vi "ADC INL_sweep_working_new.vi"(8 "error in (no error)":errorcluster, 9 "Sequence parameters":string[][](array[string])=[["Min limit", "Max limit", "Register sheet file", "Register Sheet"], ["", "", "CC2600.xls", "TX_BLE;Trim"], ["Reg write (addr;value)", "Operating frequency [Hz]", "", ""], ["NA", "2.44G", "", ""]], 10 "Run type":i32, 11 "Method parameters":T4={"Dev"={"Do not disturb DUT"=FALSE, "XOSC"=32000000.0, "Board type"="", "EM"="", "Configure tempboard"=TRUE, "Device specific info"=[], "Generic Object"=refnum}, "Method"={"Run type"=1, "Test name"="Current LPM2 4", "Comment"="", "Results folder"="", "AFC"=enum."Off", "Method name"="Current LPM2 4", "Method results"={"Excel brief report"=FALSE, "Spotfire report"=FALSE, "Starfish report"=FALSE}, "Operator"="", "Reference time"=timestamp(0 s since 1904-01-01), "AFC delay"=0.0, "Initialization"=enum."Enabled", "MD5 Sum"="", "HW addon board"=enum."None", "AFC Regsheet"="", "AFC Regfile"=path "", "dummy"=0.0}, "Inst"={"Instr"={"PS1"={"Name"="", "GPIB address"="", "VISA session"=""}, "PS2"={"Name"="", "GPIB address"="", "VISA session"=""}, "TC1"={"Name"="", "GPIB address"="", "VISA session"=""}, "TC2"={"Name"="", "GPIB address"="", "VISA session"=""}, "SA1"={"Name"="", "GPIB address"="", "VISA session"=""}, "SA2"={"Name"="", "GPIB address"="", "VISA session"=""}, "SG1"={"Name"="", "GPIB address"="", "VISA session"=""}, "SG2"={"Name"="", "GPIB address"="", "VISA session"=""}, "SG3"={"Name"="", "GPIB address"="", "VISA session"=""}, "MI1"={"Name"="", "GPIB address"="", "VISA session"=""}, "MI2"={"Name"="", "GPIB address"="", "VISA session"=""}, "SW SA"={"Name"="", "Controller addr"=""}, "SW SG"={"Name"="", "Controller addr"=""}, "MI3"={"Name"="", "GPIB address"="", "VISA session"=""}}, "Switchbox"={"RF Path"=0, "Cal compensation"=enum."TX", "Switchbox gain mode"="", "State"=enum."TX"}, "Instr to control (i.e. SA1)"="Default", "Intrument info string"=""}, "Sequence parameters"=[["Weight", "Min Limit", "Max Limit", "Register Sheet", "", "", "", "", "", "", "", "", ""], ["Vital", "", "1", "LPM2", "", "", "", "", "", "", "", "", ""], ["Resolution", "Reg write (addr;value)", "Chip mode", "Range", "", "", "", "", "", "", "", "", ""], ["u", "NA", "", "auto", "", "", "", "", "", "", "", "", ""]], "Cond"={"Temp logged"=25.0, "VDD1_PS1_6V"=-999.0, "VDD2_PS1_25V"=-999.0, "VDD4_PS2_25V"=-999.0, "VDD3_PS2_6V"=-999.0}, "Meas config"={"X-axis inner loop index"=32000000, "Y-axis outer loop index"=32000000, "X-axis"=[], "Y-axis"=[], "X-axis array req size"=32000000, "Y-axis array req size"=32000000, "Param description"=[], "Use meas clust for reporting"=FALSE, "Parameter index (page)"=0, "X-axis name"="", "Y-axis name"=""}} {"Cond"."VDD3_PS2_6V" format="%.3f"; "Cond"."VDD4_PS2_25V" format="%.3f"; "Cond"."VDD2_PS1_25V" format="%.3f"; "Cond"."VDD1_PS1_6V" format="%.3f"; "Method"."dummy" format="%.1p"; "Method"."AFC delay" format="%.1p"; "Dev"."XOSC" format="%.3p"}) -> (0 "error out":errorcluster, 1 "End method error":T3, 2 "Short Results":string[](array[string])=["0.00", "0.00", "0.00", "0.00"], 3 "Result summary":string[][](array[string])=[["Critical", "Output Power@2405 MHz", "-3", "4", "dBm"], ["Critical", "Output Power@2410 MHz", "-3", "4", "dBm"]])   [LabVIEW 2019]
doc: "[AutoDocStart]Performs crystal accuracy measurements. Measures the offset from ideal frequency. Primarily used for tuning XOSC capacitors and verifying XOSC trims.\n\nSweeping parameters: operating frequency, OSC override value and VDDR level\n\nResults: Offset frequency in ppm[AutoDocEnd]"
uses:
  User Lib/Utilities/Cluster definitions/Method input.ctl
  User Lib/Utilities/Cluster definitions/Device specific info.ctl
  User Lib/Utilities/Controls/Automatic Frequency Compensation types.ctl
  User Lib/Utilities/Controls/Method Reports.ctl
  User Lib/Utilities/Cluster definitions/Method Initialization.ctl
  User Lib/Utilities/Controls/HW addon boards.ctl
  User Lib/Utilities/Cluster definitions/Instr clust.ctl
  User Lib/Utilities/Switchbox control/SwitchBox_State._ENUMctl.ctl
  User Lib/Utilities/Cluster definitions/End method error cluster.ctl
  User Lib/Utilities/Cluster definitions/DUT vdd control.ctl
  User Lib/Utilities/Cluster definitions/DUT VDD4.ctl
  User Lib/Utilities/Cluster definitions/DUT VDD3.ctl
  User Lib/Utilities/Cluster definitions/DUT VDD2.ctl
  User Lib/Utilities/Cluster definitions/DUT VDD1.ctl
  ad5dbd7b-cdfb-4125-adc4-1165e2874c87.vi
  3f8b4189-43b3-45b7-8bba-bb7e10ae7045.vi
  42f514b6-df04-40b6-a03b-a487344522a2.vi
  dbdc58e7-b514-4632-b463-1ba2de0afab7.vi
  5201a9fb-abbc-4d1d-b83d-08253667edc6.vi
panel:
  out "output cluster 8":T1={"Average Hits \nper Code "=198.76479217603912, "Min DNL"=-0.30764433555407467, "Min INL"=-0.5231398172109945, "Max INL"=0.7801825995135989, "Max DNL"=0.8022935268616486, "DNL Range"=0.5549689312078616, "INL Range"=0.6516612083622967}
  out "ADC samples 8":u32[](array[numeric])
  out "output cluster 7":T1={"Average Hits \nper Code "=198.76479217603912, "Min DNL"=-0.30764433555407467, "Min INL"=-0.5231398172109945, "Max INL"=0.7801825995135989, "Max DNL"=0.8022935268616486, "DNL Range"=0.5549689312078616, "INL Range"=0.6516612083622967}
  out "ADC samples 7":u32[](array[numeric])
  out "output cluster 5":T1={"Average Hits \nper Code "=198.76479217603912, "Min DNL"=-0.30764433555407467, "Min INL"=-0.5231398172109945, "Max INL"=0.7801825995135989, "Max DNL"=0.8022935268616486, "DNL Range"=0.5549689312078616, "INL Range"=0.6516612083622967}
  out "ADC samples 5":u32[](array[numeric])
  in  "Tab Control":T2(tab)
  # "°C"
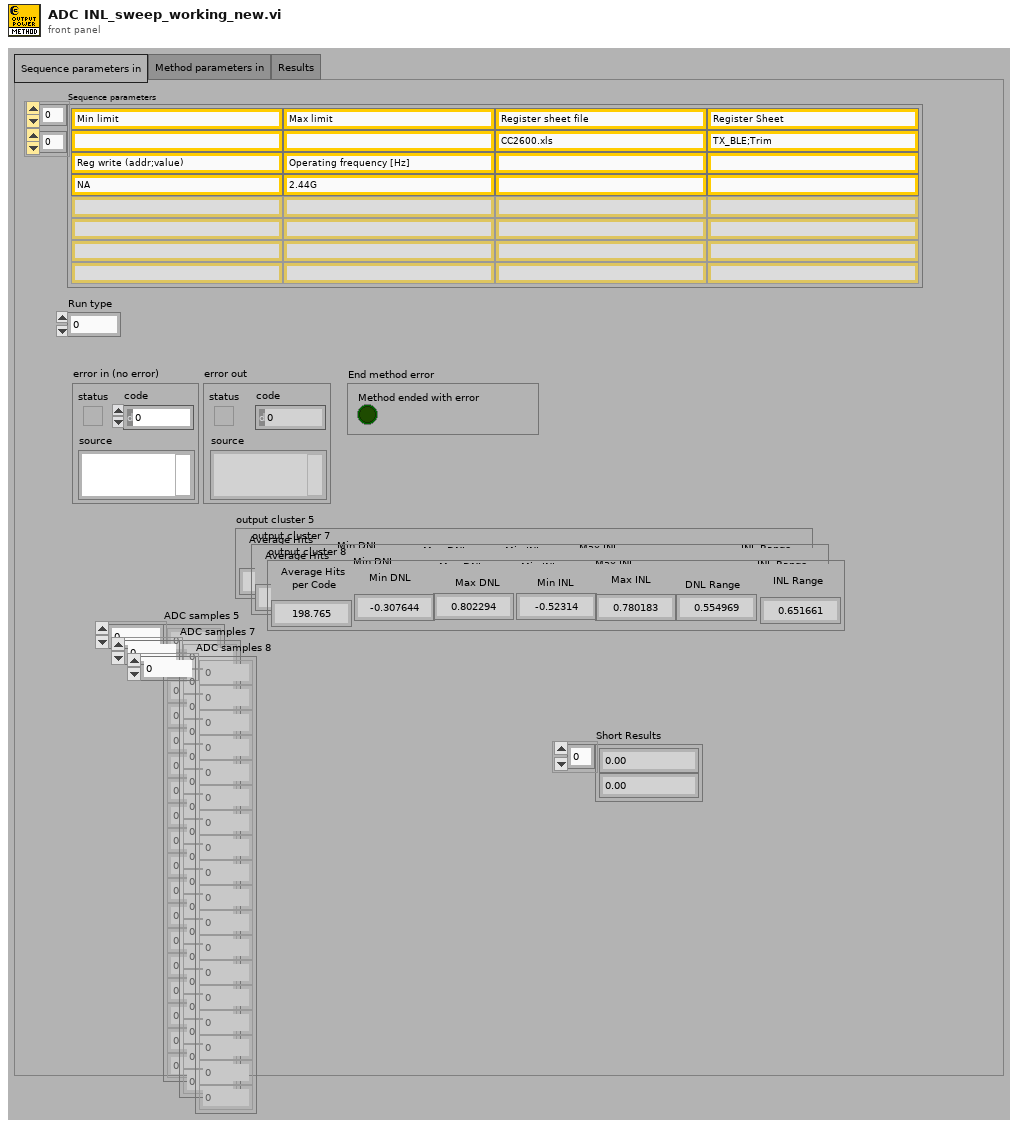
[diagram p1: front panel]
types:
  T1 = cluster{"Average Hits \nper Code ":dbl, "Min DNL":dbl, "Min INL":dbl, "Max INL":dbl, "Max DNL":dbl, "DNL Range":dbl, "INL Range":dbl}
  T2 = enum32{"Sequence parameters in", "Method parameters in", "Results"}
  T3 = typedef "End method error cluster.ctl" = cluster{"Method ended with error":bool}
  T4 = typedef "Method input.ctl" = cluster{"Dev":cluster{"Do not disturb DUT":bool, "XOSC":dbl, "Board type":string, "EM":string, "Configure tempboard":bool, "Device specific info":T5[], "Generic Object":refnum<class>}, "Method":cluster{"Run type":i32, "Test name":string, "Comment":string, "Results folder":string, "AFC":T6, "Method name":string, "Method results":T7, "Operator":string, "Reference time":timestamp, "AFC delay":dbl, "Initialization":T8, "MD5 Sum":string, "HW addon board":T9, "AFC Regsheet":string, "AFC Regfile":path, "dummy":dbl}, "Inst":T10, "Sequence parameters":string[][], "Cond":cluster{"Temp logged":dbl, "VDD1_PS1_6V":dbl, "VDD2_PS1_25V":dbl, "VDD4_PS2_25V":dbl, "VDD3_PS2_6V":dbl}, "Meas config":cluster{"X-axis inner loop index":i32, "Y-axis outer loop index":i32, "X-axis":string[], "Y-axis":string[], "X-axis array req size":i32, "Y-axis array req size":i32, "Param description":string[][], "Use meas clust for reporting":bool, "Parameter index (page)":i32, "X-axis name":string, "Y-axis name":string}}
  T5 = typedef "Device specific info.ctl" = cluster{"EM number":u8, "IP address":string, "Enabled":bool, "Slot no":u8, "RF path":u8, "EM name":string, "Wafer info":string, "AFC frequency ppm":dbl, "Register writes":string[][], "Meas data":string[][][], "Device comment":string}
  T6 = typedef "Automatic Frequency Compensation types.ctl" = enum16{"Off", "Compensate Instrument frequency", "Compensate DUT frequency", "Predictive - Compensate Instrument frequency", "Predictive - Compensate DUT frequency", "Do not skip re-init - Compensate Instrument frequency", "Do not skip re-init - Compensate DUT frequency"}
  T7 = typedef "Method Reports.ctl" = cluster{"Excel brief report":bool, "Spotfire report":bool, "Starfish report":bool}
  T8 = typedef "Method Initialization.ctl" = enum16{"Enabled", "Skip Instr and Device Init", "Enabled with Separate Flash", "Set PS, Device Init and Skip Instr Init", "Skip Device Init"}
  T9 = typedef "HW addon boards.ctl" = enum16{"None", "Current meas 5EM", "Stresstest 10EM"}
  T10 = typedef "Instr clust.ctl" = cluster{"Instr":cluster{"PS1":cluster{"Name":string, "GPIB address":string, "VISA session":refnum<visa-resource-name>}, "PS2":cluster{"Name":string, "GPIB address":string, "VISA session":refnum<visa-resource-name>}, "TC1":cluster{"Name":string, "GPIB address":string, "VISA session":refnum<visa-resource-name>}, "TC2":cluster{"Name":string, "GPIB address":string, "VISA session":refnum<visa-resource-name>}, "SA1":cluster{"Name":string, "GPIB address":string, "VISA session":refnum<visa-resource-name>}, "SA2":cluster{"Name":string, "GPIB address":string, "VISA session":refnum<visa-resource-name>}, "SG1":cluster{"Name":string, "GPIB address":string, "VISA session":refnum<visa-resource-name>}, "SG2":cluster{"Name":string, "GPIB address":string, "VISA session":refnum<visa-resource-name>}, "SG3":cluster{"Name":string, "GPIB address":string, "VISA session":refnum<visa-resource-name>}, "MI1":cluster{"Name":string, "GPIB address":string, "VISA session":refnum<visa-resource-name>}, "MI2":cluster{"Name":string, "GPIB address":string, "VISA session":refnum<visa-resource-name>}, "SW SA":cluster{"Name":string, "Controller addr":string}, "SW SG":cluster{"Name":string, "Controller addr":string}, "MI3":cluster{"Name":string, "GPIB address":string, "VISA session":refnum<visa-resource-name>}}, "Switchbox":cluster{"RF Path":i32, "Cal compensation":enum16{"TX", "RX", "Interferer", "No compensation", "Interferer2"}, "Switchbox gain mode":string, "State":T11}, "Instr to control (i.e. SA1)":string, "Intrument info string":string}
  T11 = typedef "SwitchBox_State._ENUMctl.ctl" = enum16{"TX", "RX", "SP:TX", "SP:RX", "SW:TX", "SW:RX"}
  T12 = typedef "DUT vdd control.ctl" = cluster{"VDD4 config":T13, "VDD3 config":T14, "VDD2 config":T15, "VDD1 config":T16}
  T13 = typedef "DUT VDD4.ctl" = u16
  T14 = typedef "DUT VDD3.ctl" = u16
  T15 = typedef "DUT VDD2.ctl" = u16
  T16 = typedef "DUT VDD1.ctl" = u16
  T17 = enum32{"NI Card Settings", "Memory Read Setting", "DC Capture", "ADC Ramp", "ADC Sine", "SNR", "Cap Calibration"}
  T18 = enum32{"Read from Memory", "Read .dat file", "NI Card Capture", "None"}
  T19 = cluster{"Path to Save plot":path, "Path to Raw Data plot":path}
  T20 = cluster{"Save INL/DNL Plot(Ramp)":bool, "Save SNR Plot":bool, "Save INL/DNL Plot(Sine)":bool, "Save INL/DNL Raw Data(Ramp)":bool, "Save SNR Raw Data":bool, "Save INL/DNL Raw Data(Sine)":bool, "Save DC Raw data":bool, "Save  Raw Data(Sine)":bool}
  T21 = cluster{"Min INL":dbl, "Max INL":dbl, "Min DNL":dbl, "Max DNL":dbl, "INL Range":dbl, "DNL Range":dbl, "Avg Hits/Code":dbl}
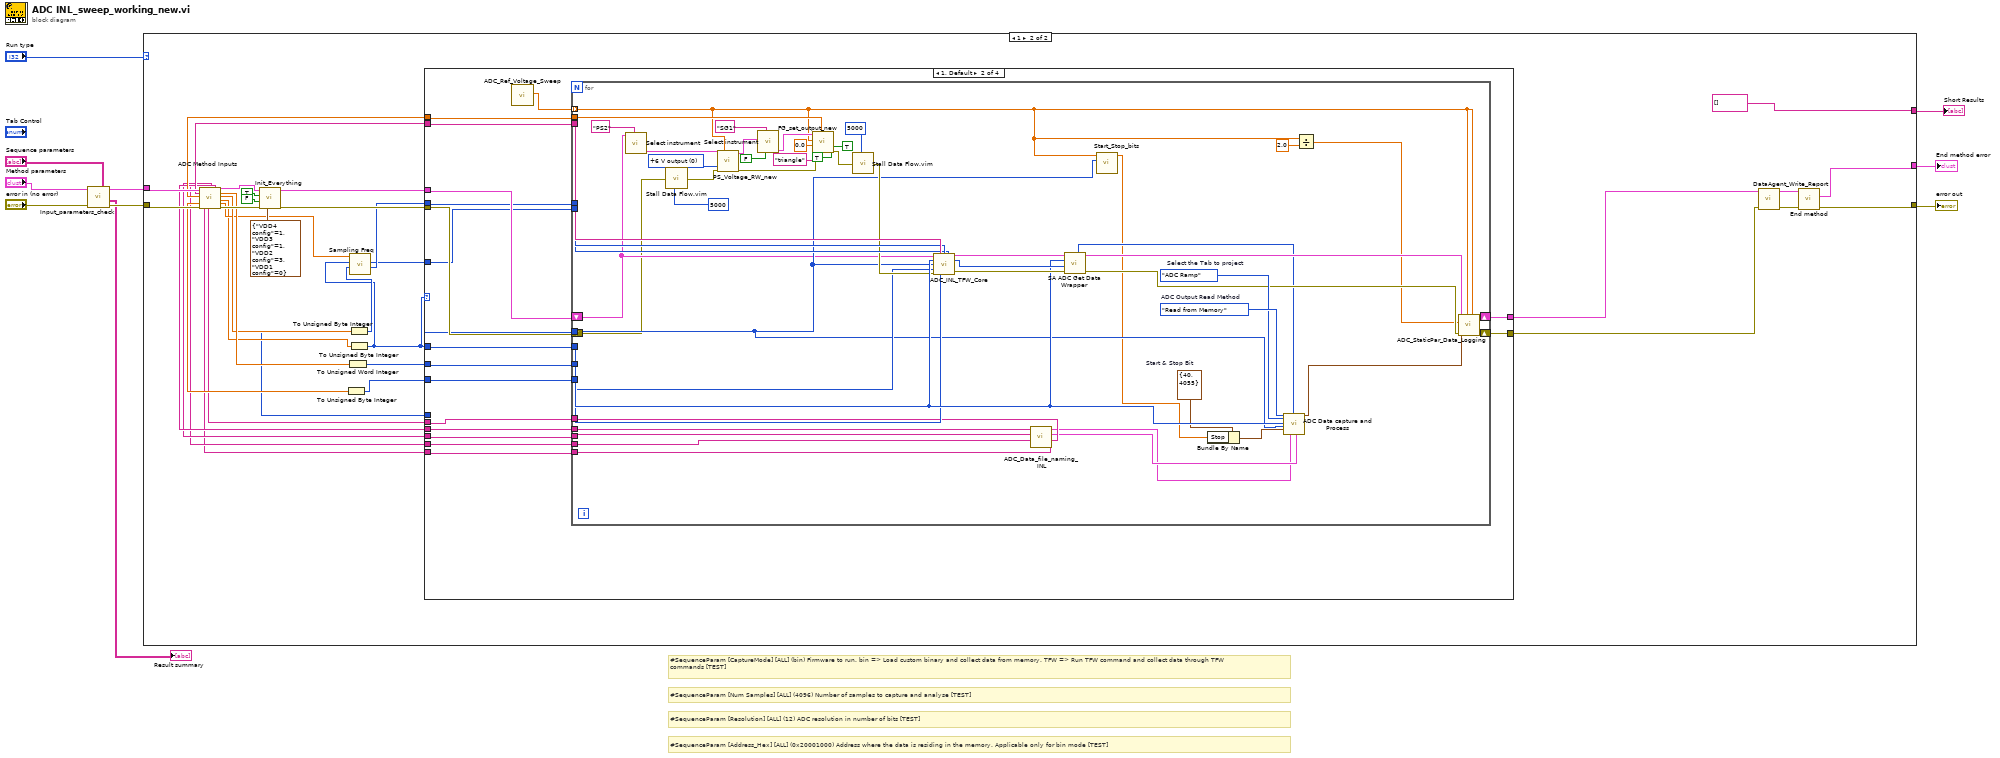
[diagram p0: block diagram]
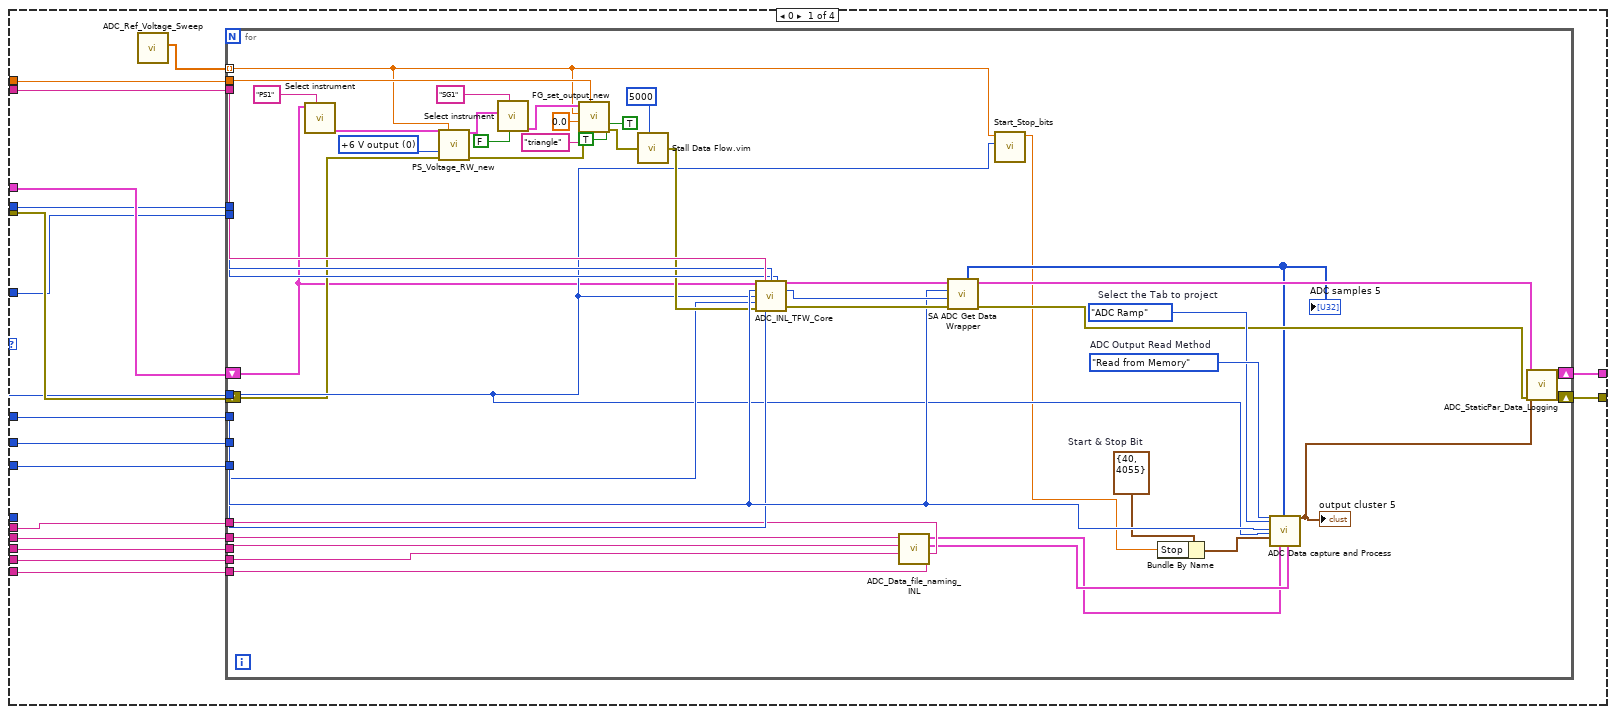
[diagram p3: hidden frame]
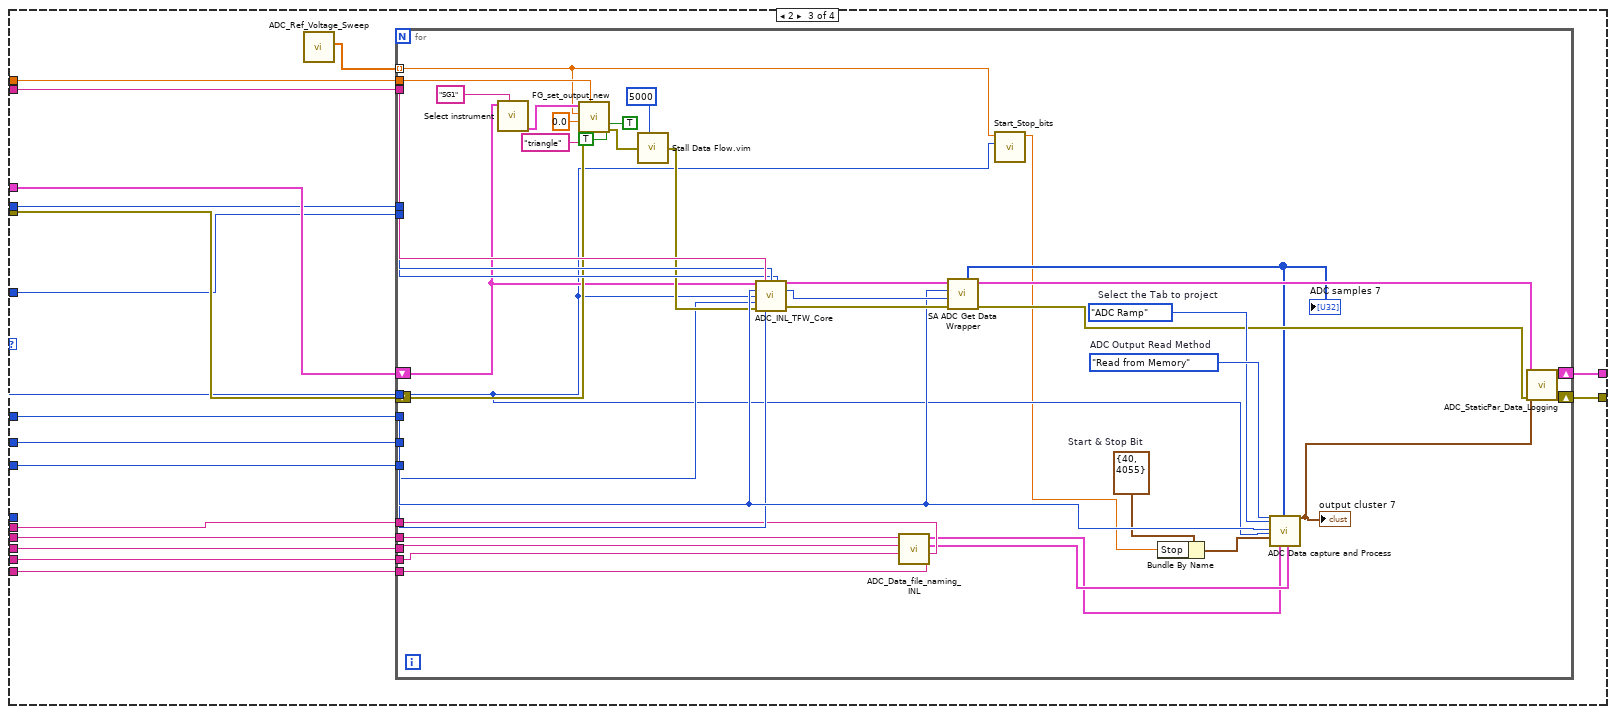
[diagram p4: hidden frame]
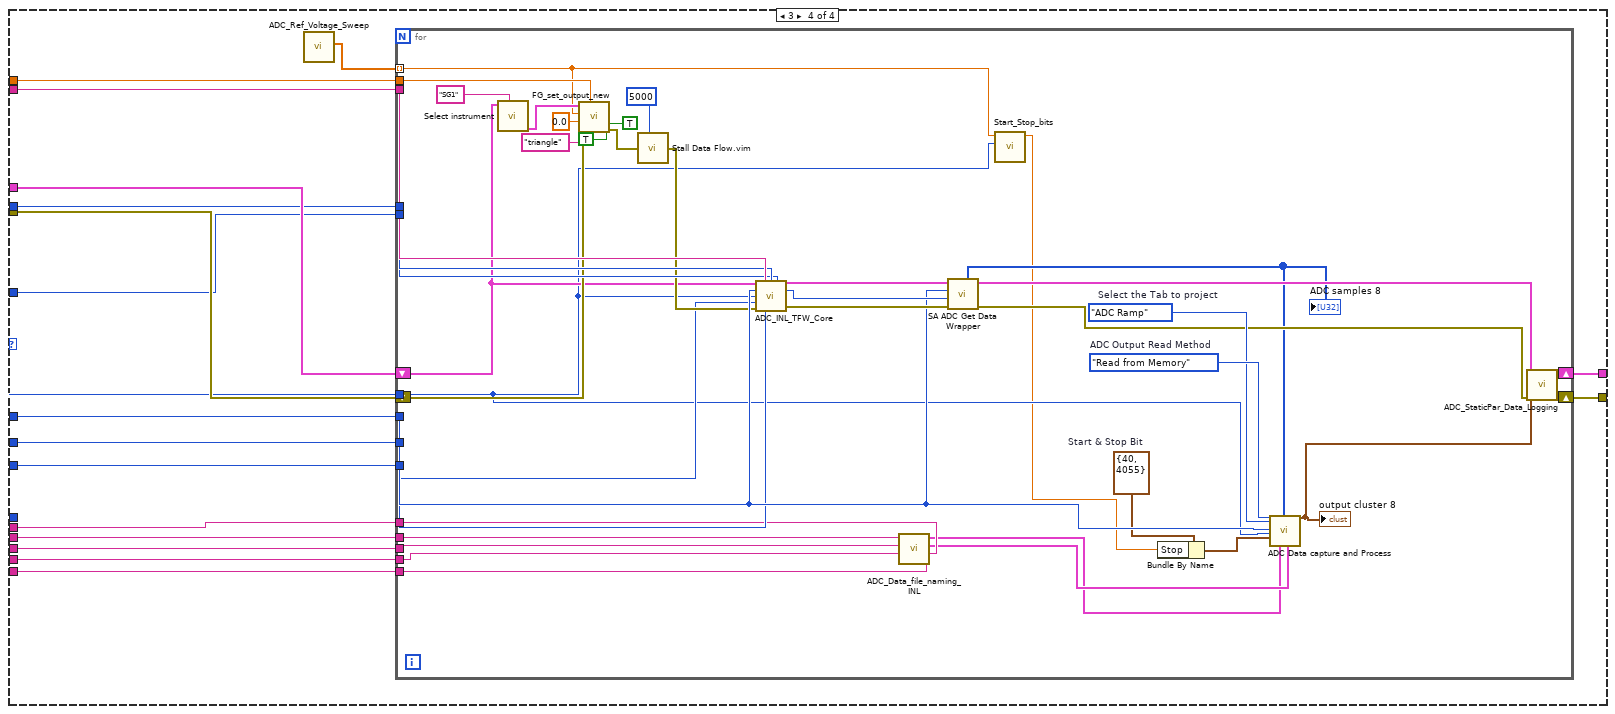
[diagram p5: hidden frame]
diagram:
  # "#SequenceParam [Num Samples] [ALL] (4096) Number of samples to capture and analyse [TEST]"
  # "#SequenceParam [CaptureMode] [ALL] (bin) Firmware to run. bin => Load custom binary and collect data from memory. TFW => Run TFW command and collect data through TFW commands [TEST]"
  # "#SequenceParam [Address_Hex] [ALL] (0x20001000) Address where the data is residing in the memory. Applicable only for bin mode [TEST]"
  # "#SequenceParam [Resolution] [ALL] (12) ADC resolution in number of bits [TEST]"
  n1 = call "Input_parameters_check.vi"("Sequence parameters"="Sequence parameters", "error in"="error in (no error)", "Method cluster in"="Method parameters") -> ("error out"=w9:errorcluster, "Result summary"=→"Result summary":string[][], "Method cluster out"=w5:T4)  [unwired: 6 in]
  n2 = case shown="1" "Run type" {
    tunnel: w9 -> [w11 w34]
    tunnel: [w11 w45] -> w10
    tunnel: w5 -> [_ w35]
    tunnel: [_ w44] -> w4
    tunnel: [_ string[] []] -> w1
    frame 0, Default {
      # "Run type 0 is only for formatting the result summary"
    }
    frame 1 {
      n3 = call "ADC Method Inputs.vi"("Method cluster in"=w35, "error in (no error)"=w34) -> ("Capture Mode"=w22:string, "Signal Freq"=w18:dbl, "ADC Chnl No."=w27:dbl, "Input Voltage String"=w14:string, "Sampling Freq String"=w15:string, "Chnl No. string"=w13:string, "Resolution String"=w16:string, "Voltage Ref String"=w17:string, "Method cluster out"=w32:T4, "Num Samples"=w31:dbl, "Resolution"=w30:dbl, "Voltage Ref"=w28:dbl, "Sampling Freq"=w29:dbl, "error out"=w33:errorcluster)  [unwired: 2 in, 2 out]
      n4 = call "Init_Everything.vi"("VDD config"=T12 {"VDD4 config"=1, "VDD3 config"=1, "VDD2 config"=3, "VDD1 config"=0}, "error in"=w33, "Support current measurement?"=FALSE, "Override VDD Config"=TRUE, "Method cluster In"=w32) -> ("error out"=w26:errorcluster, "Method cluster out"=w12:T4)  [unwired: 3 in, 2 out]
      n5 = To Unsigned Byte Integer(number=w27) -> (unsigned 8bit integer=w23:u8)
      n6 = To Unsigned Word Integer(number=w31) -> (unsigned 16bit integer=w25:u16)
      n7 = To Unsigned Byte Integer(number=w30) -> (unsigned 8bit integer=w24:u8)
      n8 = To Unsigned Byte Integer(number=w28) -> (unsigned 8bit integer=w19:u8)
      n9 = call "Sampling Freq.vi"("Resolution"=w24, "Voltage Ref"=w19, "Sampling Freq"=w29) -> ("LGPT Count"=w21:u16, "SCOMP"=w20:u16)  [unwired: 7 in]
      n10 = case shown="1, Default" w19 {
        tunnel: [w63 w128 w197 w256] -> w39
        tunnel: [w62 w127 w196 w255] -> w38
        tunnel: w12 -> [w61 w126 w195 w254]
        tunnel: w26 -> [w60 w125 w194 w253]
        tunnel: w25 -> [w59 w124 w193 w252]
        tunnel: w24 -> [w58 w123 w192 w251]
        tunnel: w19 -> [w57 w122 w191 w250]
        tunnel: w23 -> [w56 w121 w190 w249]
        tunnel: w22 -> [w55 w120 w189 w248]
        tunnel: w21 -> [w54 w119 w188 w247]
        tunnel: w20 -> [w53 w118 w187 w246]
        tunnel: w18 -> [w51 w116 w185 w244]
        tunnel: w17 -> [w50 w115 w184 w243]
        tunnel: w16 -> [w49 w114 w183 w242]
        tunnel: w15 -> [w48 w113 w182 w241]
        tunnel: w14 -> [w47 w112 w181 w240]
        tunnel: w13 -> [w46 w111 w180 w239]
        frame 0 {
          n11 = call "ADC_Ref_Voltage_Sweep.vi"() -> ("Ref voltage sweep"=w52:dbl[])  [unwired: 11 in]
          n12 = for {
            tunnel: w59 -> [w99]
            tunnel: w58 -> [w76]
            tunnel: w57 -> [w77]
            tunnel: w56 -> [w98]
            tunnel: w55 -> [w97]
            tunnel: w54 -> [w96]
            tunnel: w53 -> [w95]
            shift-right: [w105] -> w63
            shift-left: w61 -> [w69]
            shift-right: [w104] -> w62
            shift-left: w60 -> [w71]
            tunnel: w52 -> [w64] mode=indexing
            tunnel: w51 -> [w87]
            tunnel: w50 -> [w84]
            tunnel: w49 -> [w83]
            tunnel: w48 -> [w82]
            tunnel: w47 -> [w81]
            tunnel: w46 -> [w80]
            w70 = u16 0 items=["+6 V output", "+25 V output", "-25 V output", "ALL TERM"] ("Output Terminals")
            w75 = cluster{"Start":i32, "Stop":i32} {"Start"=40, "Stop"=4055}  # Start & Stop Bit
            w109 = T17."ADC Ramp"  # Select the Tab to project
            w110 = T18."Read from Memory"  # ADC Output Read Method
            n13 = call "Select instrument.vi"("Instr.Instr to control (i.e. SA1)"="PS1", "Method cluster in"=w69) -> ("Instr out"=w68:T10)  [unwired: 7 in, 2 out]
            n14 = call "PS_Voltage_RW_new.vi"("InstrCluster in"=w68, "Set Voltage"=w64, "Output Terminals"=w70, "error in (no error)"=w71) -> ("InstrCluster out"=w67:T10, "error out"=w72:errorcluster)  [unwired: 9 in, 1 out]
            n15 = call "Select instrument.vi"("Method cluster (T) / Instr cluster (F)"=FALSE, "Instr.Instr to control (i.e. SA1)"="SG1", "Instr in"=w67) -> ("Instr out"=w94:T10)  [unwired: 6 in, 2 out]
            n16 = call "FG_set_output_new.vi"("High impedance (T)"=TRUE, "Enable Output?"=TRUE, "Function (DC, Sine, Square, Triangle, Ramp up, Ramp down, Pulse)"="triangle", "Frequency [Hz]"=w87, "error in"=w72, "Low voltage"=0.0, "High voltage (or DC)"=w64, "InstrCluster in"=w94) -> ("error out"=w92:errorcluster)  [unwired: 2 in, 1 out]
            n17 = call "Stall Data Flow.vim"("value in"=w92, "milliseconds to wait"=u32 5000) -> ("value out"=w91:errorcluster)  [unwired: 1 out]
            n18 = call "ADC_INL_TFW_Core.vi"("Method cluster in"=w69, "Capture Mode"=w97, "LGPT Count"=w96, "SCOMP"=w95, "No. Samples"=w99, "Resolution"=w76, "Voltage Ref"=w77, "error in"=w91, "ADC Chnl No."=w98) -> ("Method cluster out"=w101:T4, "ResPar[0] Data Address"=w100:u32, "error out"=w102:errorcluster)  [unwired: 3 in, 1 out]
            n19 = call "ADC_Data_file_naming_INL.vi"("Amplitude (Vpp)"=w81, "ADC Chn. No"=w80, "Sampling Freq String"=w82, "Resolution String"=w83, "Voltage Ref String"=w84) -> ("path to save"=w79:T19, "Save data"=w78:T20)  [unwired: 5 in]
            n20 = call "SA ADC Get Data Wrapper.vi"("error in"=w102, "Data Address"=w100, "Num Samples"=w99, "Method cluster in"=w101) -> ("error out"=w108:errorcluster, "output cluster"=w107:T4, "ADC samples"=w106:u32[])  [unwired: 2 in, 3 out]
            "ADC samples 5" <- w106
            n21 = call "Start_Stop_bits.vi"("Resolution"=w76, "Input Amplitude"=w64) -> ("Stop Bit"=w73:dbl)  [unwired: 9 in]
            n22 = Bundle By Name(cluster=w75, "Stop"=w73) -> (w74:cluster{"Start":i32, "Stop":i32})
            n23 = call "ADC Data capture and Process.vi"("ADC Output Read Method"=w110, "Select the Tab to project"=w109, "No.of samples"=w99, "Resolution"=w76, "Start & Stop Bit"=w74, "Save data"=w78, "Input Waveform"=w106, "path to save"=w79) -> ("Static Parameters (Ramp)"=w103:T21)  [unwired: 14 in, 5 out]
            "output cluster 5" <- w103
            n24 = call "ADC_StaticPar_Data_Logging.vi"("error in (no error)"=w108, "Static Parameters (Ramp)"=w103, "output cluster"=w107) -> ("error out"=w104:errorcluster, "Method cluster out"=w105:T4)  [unwired: 7 in]
          }
        }
        frame 1, Default {
          n25 = call "ADC_Ref_Voltage_Sweep.vi"() -> ("Ref voltage sweep"=w117:dbl[])  [unwired: 11 in]
          n26 = for {
            tunnel: w124 -> [w168]
            tunnel: w123 -> [w145]
            tunnel: w122 -> [w146]
            tunnel: w121 -> [w167]
            tunnel: w120 -> [w166]
            tunnel: w119 -> [w165]
            tunnel: w118 -> [w164]
            shift-right: [w174] -> w128
            shift-left: w126 -> [w139]
            shift-right: [w173] -> w127
            shift-left: w125 -> [w133]
            tunnel: w117 -> [w129] mode=indexing
            tunnel: w116 -> [w156]
            tunnel: w115 -> [w153]
            tunnel: w114 -> [w152]
            tunnel: w113 -> [w151]
            tunnel: w112 -> [w150]
            tunnel: w111 -> [w149]
            w140 = u16 0 items=["+6 V output", "+25 V output", "-25 V output", "ALL TERM"] ("Output Terminals")
            w144 = cluster{"Start":i32, "Stop":i32} {"Start"=40, "Stop"=4055}  # Start & Stop Bit
            w178 = T17."ADC Ramp"  # Select the Tab to project
            w179 = T18."Read from Memory"  # ADC Output Read Method
            n27 = call "Select instrument.vi"("Instr.Instr to control (i.e. SA1)"="PS2", "Method cluster in"=w139) -> ("Instr out"=w138:T10)  [unwired: 7 in, 2 out]
            n28 = call "Stall Data Flow.vim"("value in"=w133, "milliseconds to wait"=u32 5000) -> ("value out"=w134:errorcluster)  [unwired: 1 out]
            n29 = call "PS_Voltage_RW_new.vi"("InstrCluster in"=w138, "Set Voltage"=w129, "Output Terminals"=w140, "error in (no error)"=w134) -> ("InstrCluster out"=w137:T10, "error out"=w141:errorcluster)  [unwired: 9 in, 1 out]
            n30 = call "Select instrument.vi"("Method cluster (T) / Instr cluster (F)"=FALSE, "Instr.Instr to control (i.e. SA1)"="SG1", "Instr in"=w137) -> ("Instr out"=w163:T10)  [unwired: 6 in, 2 out]
            n31 = call "FG_set_output_new.vi"("High impedance (T)"=TRUE, "Enable Output?"=TRUE, "Function (DC, Sine, Square, Triangle, Ramp up, Ramp down, Pulse)"="triangle", "Frequency [Hz]"=w156, "error in"=w141, "Low voltage"=0.0, "High voltage (or DC)"=w129, "InstrCluster in"=w163) -> ("error out"=w161:errorcluster)  [unwired: 2 in, 1 out]
            n32 = call "Stall Data Flow.vim"("value in"=w161, "milliseconds to wait"=u32 5000) -> ("value out"=w160:errorcluster)  [unwired: 1 out]
            n33 = call "ADC_INL_TFW_Core.vi"("Method cluster in"=w139, "Capture Mode"=w166, "LGPT Count"=w165, "SCOMP"=w164, "No. Samples"=w168, "Resolution"=w145, "Voltage Ref"=w146, "error in"=w160, "ADC Chnl No."=w167) -> ("Method cluster out"=w170:T4, "ResPar[0] Data Address"=w169:u32, "error out"=w171:errorcluster)  [unwired: 3 in, 1 out]
            n34 = call "ADC_Data_file_naming_INL.vi"("Amplitude (Vpp)"=w150, "ADC Chn. No"=w149, "Sampling Freq String"=w151, "Resolution String"=w152, "Voltage Ref String"=w153) -> ("path to save"=w148:T19, "Save data"=w147:T20)  [unwired: 5 in]
            n35 = call "SA ADC Get Data Wrapper.vi"("error in"=w171, "Data Address"=w169, "Num Samples"=w168, "Method cluster in"=w170) -> ("error out"=w177:errorcluster, "output cluster"=w176:T4, "ADC samples"=w175:u32[])  [unwired: 2 in, 3 out]
            n36 = call "Start_Stop_bits.vi"("Resolution"=w145, "Input Amplitude"=w129) -> ("Stop Bit"=w142:dbl)  [unwired: 9 in]
            n37 = Bundle By Name(cluster=w144, "Stop"=w142) -> (w143:cluster{"Start":i32, "Stop":i32})
            n38 = call "ADC Data capture and Process.vi"("ADC Output Read Method"=w179, "Select the Tab to project"=w178, "No.of samples"=w168, "Resolution"=w145, "Start & Stop Bit"=w143, "Save data"=w147, "Input Waveform"=w175, "path to save"=w148) -> ("Static Parameters (Ramp)"=w172:T21)  [unwired: 14 in, 5 out]
            n39 = Divide(x=w129, y=2.0) -> (x/y=w130:dbl)
            n40 = call "ADC_StaticPar_Data_Logging.vi"("Offset (V)"=w130, "Amplitude (Vpp)"=w129, "Ref Voltage"=w129, "error in (no error)"=w177, "Static Parameters (Ramp)"=w172, "output cluster"=w176) -> ("error out"=w173:errorcluster, "Method cluster out"=w174:T4)  [unwired: 4 in]
          }
        }
        frame 2 {
          n41 = call "ADC_Ref_Voltage_Sweep.vi"() -> ("Ref voltage sweep"=w186:dbl[])  [unwired: 11 in]
          n42 = for {
            tunnel: w193 -> [w227]
            tunnel: w192 -> [w202]
            tunnel: w191 -> [w203]
            tunnel: w190 -> [w226]
            tunnel: w189 -> [w225]
            tunnel: w188 -> [w224]
            tunnel: w187 -> [w223]
            shift-right: [w233] -> w197
            shift-left: w195 -> [w217]
            shift-right: [w232] -> w196
            shift-left: w194 -> [w220]
            tunnel: w186 -> [w201] mode=indexing
            tunnel: w185 -> [w213]
            tunnel: w184 -> [w210]
            tunnel: w183 -> [w209]
            tunnel: w182 -> [w208]
            tunnel: w181 -> [w207]
            tunnel: w180 -> [w206]
            w200 = cluster{"Start":i32, "Stop":i32} {"Start"=40, "Stop"=4055}  # Start & Stop Bit
            w237 = T17."ADC Ramp"  # Select the Tab to project
            w238 = T18."Read from Memory"  # ADC Output Read Method
            n43 = call "Select instrument.vi"("Instr.Instr to control (i.e. SA1)"="SG1", "Method cluster in"=w217) -> ("Instr out"=w222:T10)  [unwired: 7 in, 2 out]
            n44 = call "FG_set_output_new.vi"("High impedance (T)"=TRUE, "Enable Output?"=TRUE, "Function (DC, Sine, Square, Triangle, Ramp up, Ramp down, Pulse)"="triangle", "Frequency [Hz]"=w213, "error in"=w220, "Low voltage"=0.0, "High voltage (or DC)"=w201, "InstrCluster in"=w222) -> ("error out"=w219:errorcluster)  [unwired: 2 in, 1 out]
            n45 = call "Stall Data Flow.vim"("value in"=w219, "milliseconds to wait"=u32 5000) -> ("value out"=w218:errorcluster)  [unwired: 1 out]
            n46 = call "ADC_INL_TFW_Core.vi"("Method cluster in"=w217, "Capture Mode"=w225, "LGPT Count"=w224, "SCOMP"=w223, "No. Samples"=w227, "Resolution"=w202, "Voltage Ref"=w203, "error in"=w218, "ADC Chnl No."=w226) -> ("Method cluster out"=w229:T4, "ResPar[0] Data Address"=w228:u32, "error out"=w230:errorcluster)  [unwired: 3 in, 1 out]
            n47 = call "ADC_Data_file_naming_INL.vi"("Amplitude (Vpp)"=w207, "ADC Chn. No"=w206, "Sampling Freq String"=w208, "Resolution String"=w209, "Voltage Ref String"=w210) -> ("path to save"=w205:T19, "Save data"=w204:T20)  [unwired: 5 in]
            n48 = call "SA ADC Get Data Wrapper.vi"("error in"=w230, "Data Address"=w228, "Num Samples"=w227, "Method cluster in"=w229) -> ("error out"=w236:errorcluster, "output cluster"=w235:T4, "ADC samples"=w234:u32[])  [unwired: 2 in, 3 out]
            "ADC samples 7" <- w234
            n49 = call "Start_Stop_bits.vi"("Resolution"=w202, "Input Amplitude"=w201) -> ("Stop Bit"=w198:dbl)  [unwired: 9 in]
            n50 = Bundle By Name(cluster=w200, "Stop"=w198) -> (w199:cluster{"Start":i32, "Stop":i32})
            n51 = call "ADC Data capture and Process.vi"("ADC Output Read Method"=w238, "Select the Tab to project"=w237, "No.of samples"=w227, "Resolution"=w202, "Start & Stop Bit"=w199, "Save data"=w204, "Input Waveform"=w234, "path to save"=w205) -> ("Static Parameters (Ramp)"=w231:T21)  [unwired: 14 in, 5 out]
            "output cluster 7" <- w231
            n52 = call "ADC_StaticPar_Data_Logging.vi"("error in (no error)"=w236, "Static Parameters (Ramp)"=w231, "output cluster"=w235) -> ("error out"=w232:errorcluster, "Method cluster out"=w233:T4)  [unwired: 7 in]
          }
        }
        frame 3 {
          n53 = call "ADC_Ref_Voltage_Sweep.vi"() -> ("Ref voltage sweep"=w245:dbl[])  [unwired: 11 in]
          n54 = for {
            tunnel: w252 -> [w286]
            tunnel: w251 -> [w261]
            tunnel: w250 -> [w262]
            tunnel: w249 -> [w285]
            tunnel: w248 -> [w284]
            tunnel: w247 -> [w283]
            tunnel: w246 -> [w282]
            shift-right: [w292] -> w256
            shift-left: w254 -> [w276]
            shift-right: [w291] -> w255
            shift-left: w253 -> [w279]
            tunnel: w245 -> [w260] mode=indexing
            tunnel: w244 -> [w272]
            tunnel: w243 -> [w269]
            tunnel: w242 -> [w268]
            tunnel: w241 -> [w267]
            tunnel: w240 -> [w266]
            tunnel: w239 -> [w265]
            w259 = cluster{"Start":i32, "Stop":i32} {"Start"=40, "Stop"=4055}  # Start & Stop Bit
            w296 = T17."ADC Ramp"  # Select the Tab to project
            w297 = T18."Read from Memory"  # ADC Output Read Method
            n55 = call "Select instrument.vi"("Instr.Instr to control (i.e. SA1)"="SG1", "Method cluster in"=w276) -> ("Instr out"=w281:T10)  [unwired: 7 in, 2 out]
            n56 = call "FG_set_output_new.vi"("High impedance (T)"=TRUE, "Enable Output?"=TRUE, "Function (DC, Sine, Square, Triangle, Ramp up, Ramp down, Pulse)"="triangle", "Frequency [Hz]"=w272, "error in"=w279, "Low voltage"=0.0, "High voltage (or DC)"=w260, "InstrCluster in"=w281) -> ("error out"=w278:errorcluster)  [unwired: 2 in, 1 out]
            n57 = call "Stall Data Flow.vim"("value in"=w278, "milliseconds to wait"=u32 5000) -> ("value out"=w277:errorcluster)  [unwired: 1 out]
            n58 = call "ADC_INL_TFW_Core.vi"("Method cluster in"=w276, "Capture Mode"=w284, "LGPT Count"=w283, "SCOMP"=w282, "No. Samples"=w286, "Resolution"=w261, "Voltage Ref"=w262, "error in"=w277, "ADC Chnl No."=w285) -> ("Method cluster out"=w288:T4, "ResPar[0] Data Address"=w287:u32, "error out"=w289:errorcluster)  [unwired: 3 in, 1 out]
            n59 = call "ADC_Data_file_naming_INL.vi"("Amplitude (Vpp)"=w266, "ADC Chn. No"=w265, "Sampling Freq String"=w267, "Resolution String"=w268, "Voltage Ref String"=w269) -> ("path to save"=w264:T19, "Save data"=w263:T20)  [unwired: 5 in]
            n60 = call "SA ADC Get Data Wrapper.vi"("error in"=w289, "Data Address"=w287, "Num Samples"=w286, "Method cluster in"=w288) -> ("error out"=w295:errorcluster, "output cluster"=w294:T4, "ADC samples"=w293:u32[])  [unwired: 2 in, 3 out]
            "ADC samples 8" <- w293
            n61 = call "Start_Stop_bits.vi"("Resolution"=w261, "Input Amplitude"=w260) -> ("Stop Bit"=w257:dbl)  [unwired: 9 in]
            n62 = Bundle By Name(cluster=w259, "Stop"=w257) -> (w258:cluster{"Start":i32, "Stop":i32})
            n63 = call "ADC Data capture and Process.vi"("ADC Output Read Method"=w297, "Select the Tab to project"=w296, "No.of samples"=w286, "Resolution"=w261, "Start & Stop Bit"=w258, "Save data"=w263, "Input Waveform"=w293, "path to save"=w264) -> ("Static Parameters (Ramp)"=w290:T21)  [unwired: 14 in, 5 out]
            "output cluster 8" <- w290
            n64 = call "ADC_StaticPar_Data_Logging.vi"("error in (no error)"=w295, "Static Parameters (Ramp)"=w290, "output cluster"=w294) -> ("error out"=w291:errorcluster, "Method cluster out"=w292:T4)  [unwired: 7 in]
          }
        }
      }
      n65 = call "DataAgent_Write_Report.vi"("error in (no error)"=w38, "Method cluster in"=w39) -> ("error out"=w42:errorcluster, "Method cluster out"=w41:T4)  [unwired: 8 in]
      n66 = call "End method.vi"("error in"=w42, "Method cluster in"=w41) -> ("error out"=w45:errorcluster, "End method error"=w44:T3)  [unwired: 7 in, 1 out]
    }
  }
  "error out" <- w10
  "End method error" <- w4
  "Short Results" <- w1
